vi "RejectNSigmaOutliers.vi"(9 "Repeat Until Clean (F: Run Once)":bool, 10 "N Sigma":dbl, 11 "Cluster in":cluster{dbl[], dbl[]}) -> (1 "Nothing Rejected":bool, 2 "Sigma":dbl format="%0.2f", 3 "Cluster out":cluster{dbl[], dbl[]}, 4 "N Loops":i16, 5 "N Rejected":i16)   [LabVIEW 2019]
uses:
  <vilib>/Analysis/NI_AALBase.lvlib
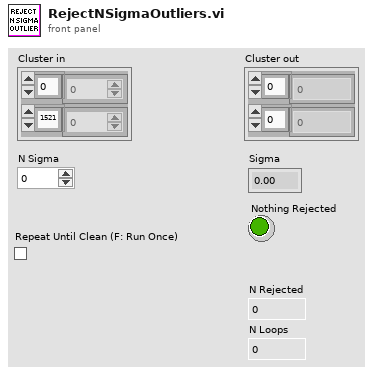
[diagram p1: front panel]
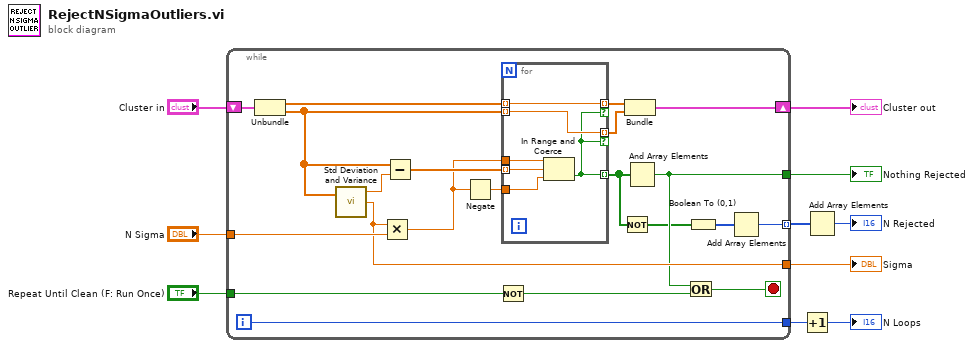
[diagram p0: block diagram]
diagram:
  n1 = while {
    tunnel: "N Sigma" -> [w26]
    tunnel: [w23] -> w7
    tunnel: [w25] -> w6
    shift-right: [w29] -> w9
    shift-left: "Cluster in" -> [w30]
    tunnel: "Repeat Until Clean (F: Run Once)" -> [w22]
    tunnel: [w19] -> w4
    tunnel: [w15] -> w3 mode=indexing
    i -> [w19]
    stop <- w20 stop-if-true
    n2 = Unbundle(w30) -> (w11:dbl[], w31:dbl[])
    n3 = call <vilib>:"Std Deviation and Variance.vi"("X"=w31) -> ("mean"=w24:dbl, "standard deviation"=w25:dbl)  [unwired: 1 in, 1 out]
    n4 = Multiply(x=w25, y=w26) -> (x*y=w12:dbl)
    n5 = Subtract(x=w31, y=w24) -> (x-y=w14:dbl[])
    n6 = Negate(x=w12) -> (-x=w13:dbl)
    n7 = Not(x=w22) -> (.not. x?=w21:bool)
    n8 = for {
      tunnel: w11 -> [w36] mode=indexing
      tunnel: w31 -> [w35] mode=indexing
      tunnel: w14 -> [w37] mode=indexing
      tunnel: [w36] -> w27 mode=indexing if=w34
      tunnel: [w35] -> w28 mode=indexing if=w34
      tunnel: [w34] -> w18 mode=indexing
      tunnel: w13 -> [w33]
      tunnel: w12 -> [w32]
      n9 = In Range and Coerce(upper limit=w32, x=w37, lower limit=w33) -> (In Range?=w34:bool)  [unwired: 1 out]
    }
    n10 = Not(x=w18) -> (.not. x?=w17:bool[])
    n11 = Bundle(w27, w28) -> (w29:cluster{dbl[], dbl[]})  [unwired: 1 in]
    n12 = And Array Elements(Boolean array=w18) -> (logical AND=w23:bool)
    n13 = Or(x=w23, y=w21) -> (x .or. y?=w20:bool)
    n14 = Boolean To (0,1)(Boolean=w17) -> (0, 1=w16:i16[])
    n15 = Add Array Elements(numeric array=w16) -> (sum=w15:i16)
  }
  "Sigma" <- w6
  "Cluster out" <- w9
  "Nothing Rejected" <- w7
  n16 = Increment(x=w4) -> (x+1=→"N Loops":i32)
  n17 = Add Array Elements(numeric array=w3) -> (sum=→"N Rejected":i16)
